vi "guess.vi"() -> ()   [LabVIEW 2016]
uses:
  <vilib>/Utility/file.llb/Write To Spreadsheet File (string).vi
panel:
  out "appended array":string[][](array[string])
  out "Column Header Strings[]":string[](array[string])
  out "Item Names":string[][](array[string])
  in  "Work Space  information":i32(listbox)
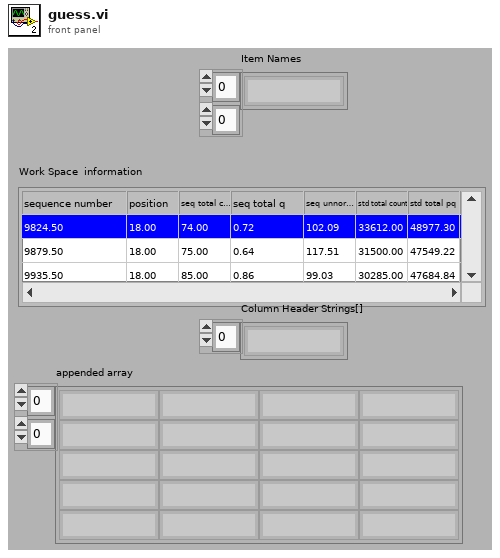
[diagram p1: front panel]
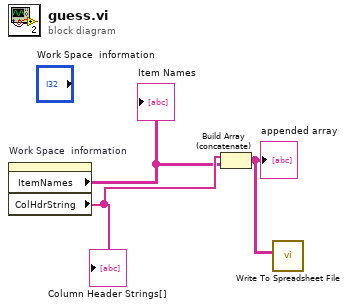
[diagram p0: block diagram]
diagram:
  n1 = property on="Work Space  information" class="MCListbox (strict)"() -> ("ItemNames"=w2:string[][], "ColHdrString"=w3:string[])  [unwired: 2 in, 2 out]
  "Item Names" <- w2
  "Column Header Strings[]" <- w3
  n2 = Build Array (concatenate)(w3, w2) -> (w1:string[][])
  "appended array" <- w1
  n3 = call-poly <vilib>:"Write To Spreadsheet File.vi"("2D data"=w1) -> ()  [unwired: 7 in, 1 out]
